vi "error_not_supported_storage_mode.vi"(8 "error in (no error)":errorcluster, 11 "ImageCollection in":refnum<class "ImageCollection.lvclass">) -> (0 "error out":errorcluster, 3 "ImageCollection out":refnum<class "ImageCollection.lvclass">)   [LabVIEW 2010, in "ImageCollection.lvclass"]
uses:
  ImageCollection.lvclass
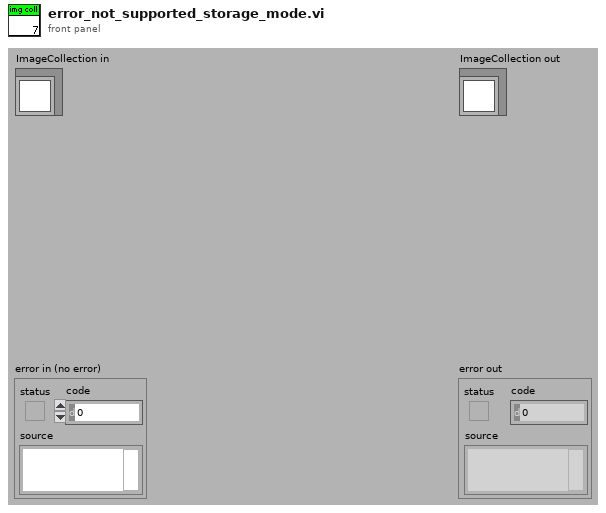
[diagram p1: front panel]
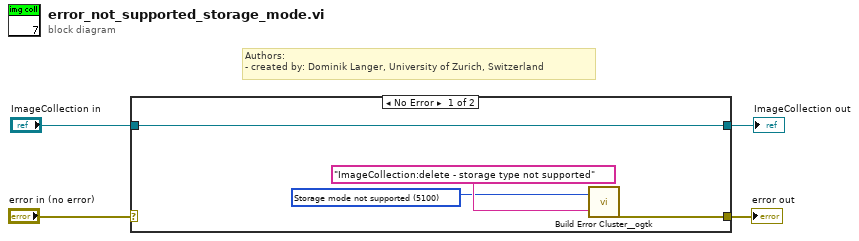
[diagram p0: block diagram]
diagram:
  # "Authors: \n- created by: Dominik Langer, University of Zurich, Switzerland"
  n1 = case shown="No Error" "error in (no error)" {
    selector: "error in (no error)" -> [_ w10]
    tunnel: [w5 w10] -> w3
    tunnel: [w8 w9] -> w1
    tunnel: "ImageCollection in" -> [w8 w9]
    frame No Error {
      w6 = u16 5100 items=["Storage mode not supported"=5100] ("Ring")
      n2 = call <userlib>:"Build Error Cluster__ogtk.vi"("String to Prepend to source (\"\")"="ImageCollection:delete - storage type not supported" ("String to Prepend to source (\"\")"), "code"=w6) -> ("error out"=w5:errorcluster)
    }
    frame Error {
    }
  }
  "error out" <- w3
  "ImageCollection out" <- w1
